vi "Zeitstempel-Array zusammenstutzen.vi"(8 "Array":timestamp[](array[timestamp]), 10 "Anzahl Elemente":i32) -> (0 "Array":timestamp[](array[timestamp]))   [LabVIEW 2013, in "allgemeine Sub-VIs.lvlib"]
uses:
  allgemeine Sub-VIs.lvlib
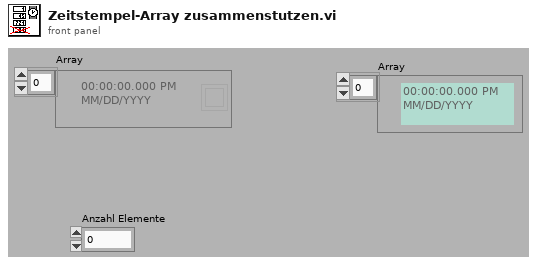
[diagram p1: front panel]
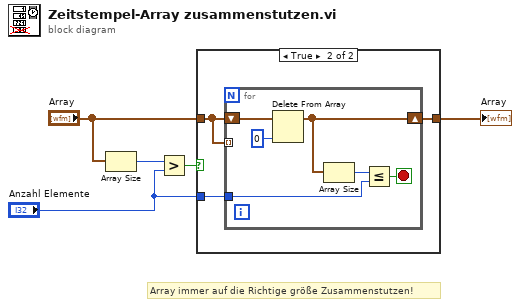
[diagram p0: block diagram]
diagram:
  # "Array immer auf die Richtige größe Zusammenstutzen!"
  n1 = Array Size(array="Array") -> (size(s)=w4:i32)
  n2 = Greater?(x=w4, y="Anzahl Elemente") -> (0:w5:bool)
  n3 = case shown="True" w5 {
    tunnel: "Array" -> [w6 w8]
    tunnel: [w6 w7] -> w1
    tunnel: "Anzahl Elemente" -> [_ w9]
    frame False {
    }
    frame True {
      n4 = for {
        tunnel: w9 -> [w14]
        tunnel: w8 -> [_] mode=indexing
        shift-right: [w10] -> w7
        shift-left: w8 -> [w11]
        stop <- w13 stop-if-true
        n5 = Delete From Array(array=w11, index=0 ("Index")) -> (array with subset deleted=w10:timestamp[])  [unwired: 1 in, 1 out]
        n6 = Array Size(array=w10) -> (size(s)=w15:i32)
        n7 = Less Or Equal?(x=w15, y=w14) -> (x <= y?=w13:bool)
      }
    }
  }
  "Array" <- w1
